vi "KeysPressed-SubVI.vi"(1 "Key values":cluster{i32, i32, i32, i32, i32, i32, i32}, 2 "device ID":refnum<k1>) -> (0 "Stop = TRUE":bool)   [LabVIEW 2014]
uses:
  <vilib>/Utility/inputDevices.llb/keyboardAcquire.vi
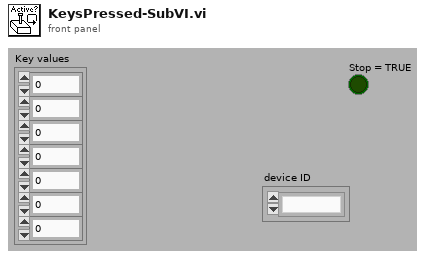
[diagram p1: front panel]
types:
  T1 = enum16{"0", "1", "2", "3", "4", "5", "6", "7", "8", "9", "A", "B", "C", "D", "E", "F", "G", "H", "I", "J", "K", "L", "M", "N", "O", "P", "Q", "R", "S", "T", "U", "V", "W", "X", "Y", "Z", "F1", "F2", "F3", "F4", "F5", "F6", "F7", "F8", "F9", "F10", "F11", "F12", "F13", "F14", "F15", "ADD", "BACK", "BACKSLASH", "CAPITAL", "COMMA", "DECIMAL", "DELETE", "DIVIDE", "DOWN", "END", "EQUALS", "ESCAPE", "GRAVE (`)", "HOME", "INSERT", "LBRACKET", "LCONTROL", "LEFT", "L ALT", "LSHIFT", "LWIN", "MINUS", "MULTIPLY", "NEXT", "NUMLOCK", "NUMPAD_0", "NUMPAD_1", "NUMPAD_2", "NUMPAD_3", "NUMPAD_4", "NUMPAD_5", "NUMPAD_6", "NUMPAD_7", "NUMPAD_8", "NUMPAD_9", "PAUSE", "PERIOD", "PRIOR (PG UP)", "RBRACKET", "RCONTROL", "RETURN", "RIGHT", "R ALT", "RSHIFT", "RWIN", "SCROLL", "SEMICOLON", "SLASH", "SPACE", "SUBTRACT", "TAB", "UP", "ENTER (num pad)", "' (quote)"}[]
  T2 = enum16{"0", "1", "2", "3", "4", "5", "6", "7", "8", "9", "A", "B", "C", "D", "E", "F", "G", "H", "I", "J", "K", "L", "M", "N", "O", "P", "Q", "R", "S", "T", "U", "V", "W", "X", "Y", "Z", "F1", "F2", "F3", "F4", "F5", "F6", "F7", "F8", "F9", "F10", "F11", "F12", "F13", "F14", "F15", "ADD", "BACK", "BACKSLASH", "CAPITAL", "COMMA", "DECIMAL", "DELETE", "DIVIDE", "DOWN", "END", "EQUALS", "ESCAPE", "GRAVE (`)", "HOME", "INSERT", "LBRACKET", "LCONTROL", "LEFT", "L ALT", "LSHIFT", "LWIN", "MINUS", "MULTIPLY", "NEXT", "NUMLOCK", "NUMPAD_0", "NUMPAD_1", "NUMPAD_2", "NUMPAD_3", "NUMPAD_4", "NUMPAD_5", "NUMPAD_6", "NUMPAD_7", "NUMPAD_8", "NUMPAD_9", "PAUSE", "PERIOD", "PRIOR (PG UP)", "RBRACKET", "RCONTROL", "RETURN", "RIGHT", "R ALT", "RSHIFT", "RWIN", "SCROLL", "SEMICOLON", "SLASH", "SPACE", "SUBTRACT", "TAB", "UP", "ENTER (num pad)", "' (quote)"}
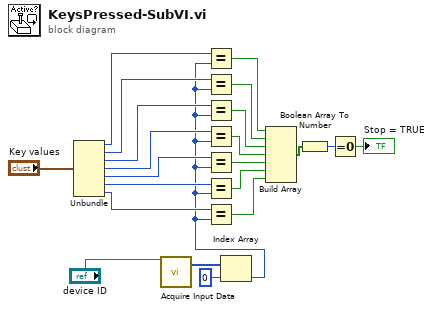
[diagram p0: block diagram]
diagram:
  n1 = Unbundle("Key values") -> (w10:i32, w9:i32, w8:i32, w7:i32, w6:i32, w5:i32, w4:i32)
  n2 = call-poly <vilib>:"Acquire Input Data.vi"("device ID"="device ID") -> ("keys pressed"=w20:T1)  [unwired: 1 in, 17 out]
  n3 = Index Array(array=w20, index=0) -> (element=w3:T2)
  n4 = Equal?(x=w10, y=w3) -> (x = y?=w16:bool)
  n5 = Equal?(x=w9, y=w3) -> (x = y?=w17:bool)
  n6 = Equal?(x=w8, y=w3) -> (x = y?=w18:bool)
  n7 = Equal?(x=w7, y=w3) -> (x = y?=w19:bool)
  n8 = Equal?(x=w6, y=w3) -> (x = y?=w12:bool)
  n9 = Equal?(x=w5, y=w3) -> (x = y?=w2:bool)
  n10 = Equal?(x=w4, y=w3) -> (x = y?=w1:bool)
  n11 = Build Array(w16, w17, w18, w19, w12, w2, w1) -> (w15:bool[])
  n12 = Boolean Array To Number(Boolean array=w15) -> (number=w14:u32)
  n13 = Equal To 0?(x=w14) -> (x = 0?=→"Stop = TRUE":bool)
